vi "Remove All.vi"(8 "error in (no error)":errorcluster, 10 "Action":T1, 11 "Custom Device reference in":refnum<k24>) -> (0 "error out":errorcluster, 3 "Custom Device reference out":refnum<k24>)   [LabVIEW 2023, in "J1939 System Definition API Support.lvlib"]
uses:
  J1939 System Definition API Support.lvlib
  NationalInstruments.VeriStand.SystemDefinitionAPI
  Types/Remove Frame Action.ctl
  Addon/Addon Shared/SubVIs/Constants.vi
  <vilib>/NI VeriStand/Custom Device Tools/Custom Device Utility Library/NI VeriStand - Search for All Items by GUID.vi
  <vilib>/NI VeriStand/Custom Device Tools/Custom Device Utility Library/Custom Device Utility Library.lvlib
  <vilib>/NI VeriStand/Custom Device API/Custom Device API.lvlib
  Addon/Addon Shared/J1939 Addon Shared.lvlib
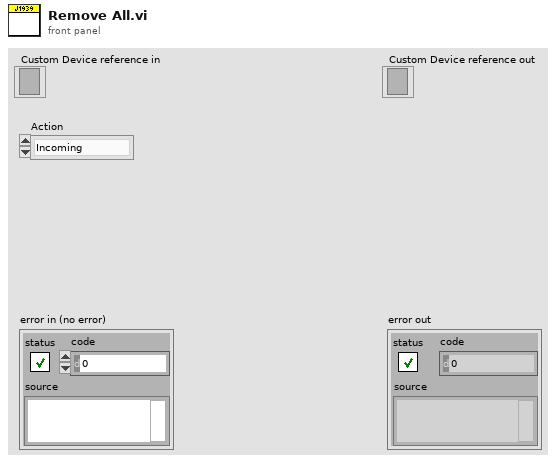
[diagram p1: front panel]
types:
  T1 = typedef "J1939 System Definition API Support.lvlib/Remove Frame Action.ctl" = enum16{"Incoming", "Outgoing Event", "Outgoing Cyclic", "Outgoing Cyclic Event"}
  T2 = typedef "Custom Device API.lvlib/Custom Device Item Ref.ctl" = u64
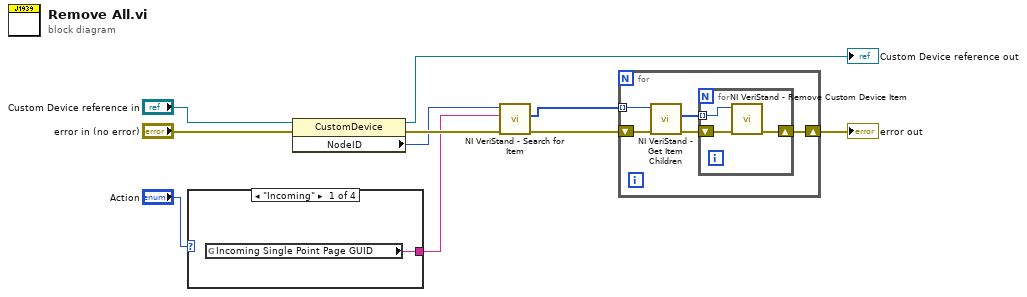
[diagram p0: block diagram]
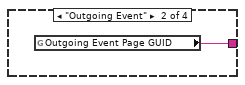
[diagram p2: hidden frame]
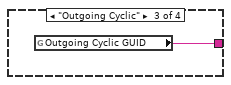
[diagram p3: hidden frame]
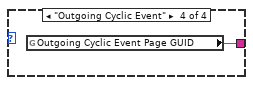
[diagram p4: hidden frame]
diagram:
  n1 = case shown="\"Incoming\"" "Action" {
    tunnel: [w11 w12 w13 w14] -> w1
    frame "Incoming" {
      n2 = global read "Constants.vi" "Incoming Single Point Page GUID"() -> (w11:string)
    }
    frame "Outgoing Event" {
      n3 = global read "Constants.vi" "Outgoing Event Page GUID"() -> (w12:string)
    }
    frame "Outgoing Cyclic" {
      n4 = global read "Constants.vi" "Outgoing Cyclic GUID"() -> (w13:string)
    }
    frame "Outgoing Cyclic Event" {
      n5 = global read "Constants.vi" "Outgoing Cyclic Event Page GUID"() -> (w14:string)
    }
  }
  n6 = property class="CustomDevice"(reference="Custom Device reference in", error in="error in (no error)") -> (reference out=→"Custom Device reference out":refnum<k24>, error out=w7:errorcluster, "NodeID"=w6:u64)
  n7 = call-poly <vilib>:"NI VeriStand - Search for Item.vi"("error in"=w7, "Item GUID"=w1, "Section Ref in"=w6) -> ("error out"=w3:errorcluster, "Item Refs"=w4:T2[])  [unwired: 5 in, 2 out]
  n8 = for {
    tunnel: w4 -> [w18] mode=indexing
    shift-right: [w19] -> w5
    shift-left: w3 -> [w16]
    n9 = call <vilib>:"NI VeriStand - Get Item Children.vi"("error in (no error)"=w16, "Item Ref in"=w18) -> ("error out"=w15:errorcluster, "Child Refs"=w17:T2[])  [unwired: 6 in, 2 out]
    n10 = for {
      tunnel: w17 -> [w20] mode=indexing
      shift-right: [w22] -> w19
      shift-left: w15 -> [w21]
      n11 = call <vilib>:"NI VeriStand - Remove Custom Device Item.vi"("error in (no error)"=w21, "Item Ref in"=w20) -> ("error out"=w22:errorcluster)  [unwired: 8 in, 1 out]
    }
  }
  "error out" <- w5
